vi "svc_Get Weighting Enum and Labels.vi"(8 "weighting filter":T1 items=["Linear", "A-weighting", "B-weighting", "C-weighting", "ITU-R 468-4", "Dolby", "CCITT", "C-message", "Wb", "Wc", "Wd", "We", "Wf", "Wh", "Wj", "Wk", "Wm", "AES17 20 kHz lowpass", "AES17 40 kHz lowpass", "AES17 20 kHz highpass", "AES17 40 kHz highpass"]) -> (1 "weighting subarray":string[](array[string]), 2 "weighting enum":T1 items=["Linear", "A-weighting", "B-weighting", "C-weighting", "ITU-R 468-4", "Dolby", "CCITT", "C-message", "Wb", "Wc", "Wd", "We", "Wf", "Wh", "Wj", "Wk", "Wm", "AES17 20 kHz lowpass", "AES17 40 kHz lowpass", "AES17 20 kHz highpass", "AES17 40 kHz highpass"])   [LabVIEW 2017]
uses:
  <vilib>/addons/_NISVFA/_Shared subVIs/Controls/svc_Weighting Filter Text Ring.ctl
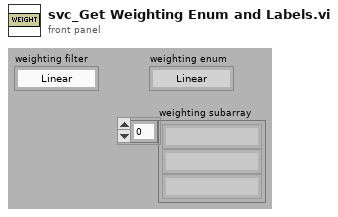
[diagram p1: front panel]
types:
  T1 = typedef "svc_Weighting Filter Text Ring.ctl" = u16
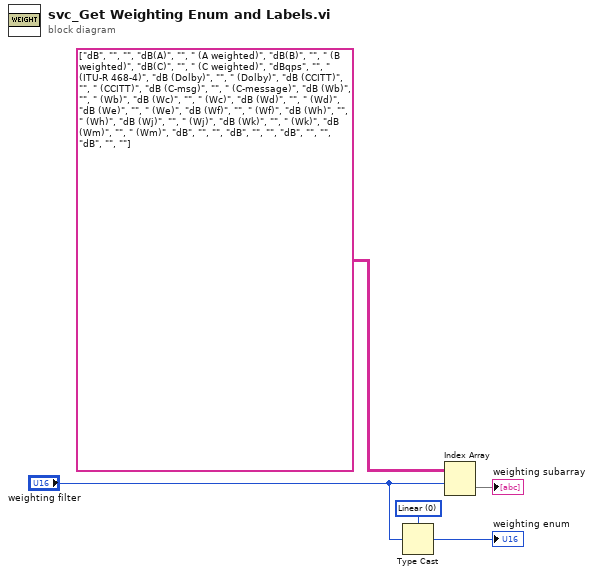
[diagram p0: block diagram]
diagram:
  w4 = T1 0 items=["Linear", "A-weighting", "B-weighting", "C-weighting", "ITU-R 468-4", "Dolby", "CCITT", "C-message", "Wb", "Wc", "Wd", "We", "Wf", "Wh", "Wj", "Wk", "Wm", "AES17 20 kHz lowpass", "AES17 40 kHz lowpass", "AES17 20 kHz highpass", "AES17 40 kHz highpass", "Undefined"] ("weighting enum")
  n1 = Type Cast(type=w4, x="weighting filter") -> (*(type *) &x=→"weighting enum":T1)
  n2 = Index Array(array=string[][] [["dB", "", ""], ["dB(A)", "", " (A weighted)"], ["dB(B)", "", " (B weighted)"], ["dB(C)", "", " (C weighted)"], ["dBqps", "", " (ITU-R 468-4)"], ["dB (Dolby)", "", " (Dolby)"], ["dB (CCITT)", "", " (CCITT)"], ["dB (C-msg)", "", " (C-message)"], ["dB (Wb)", "", " (Wb)"], ["dB (Wc)", "", " (Wc)"], ["dB (Wd)", "", " (Wd)"], ["dB (We)", "", " (We)"], ["dB (Wf)", "", " (Wf)"], ["dB (Wh)", "", " (Wh)"], ["dB (Wj)", "", " (Wj)"], ["dB (Wk)", "", " (Wk)"], ["dB (Wm)", "", " (Wm)"], ["dB", "", ""], ["dB", "", ""], ["dB", "", ""], ["dB", "", ""]] ("transposed array"), index (row)="weighting filter") -> (element=→"weighting subarray":string[])  [unwired: 1 in]
